vi "LogFile.vi"(7 "LogMode":T1, 8 "error in (no error)":errorcluster, 11 "LogString":string="456") -> (0 "error out":errorcluster)   [LabVIEW 2011]
uses:
  Enumerator/LogMode.ctl
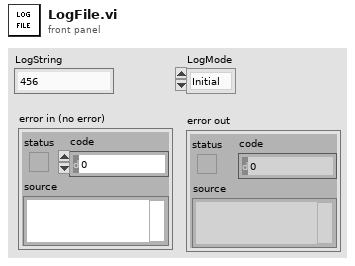
[diagram p1: front panel]
types:
  T1 = typedef "LogMode.ctl" = enum16{"Initial", "Creat", "Write", "Close"}
  T2 = enum16{"open", "replace", "create", "open or create", "replace or create", "replace or create with confirmation"}
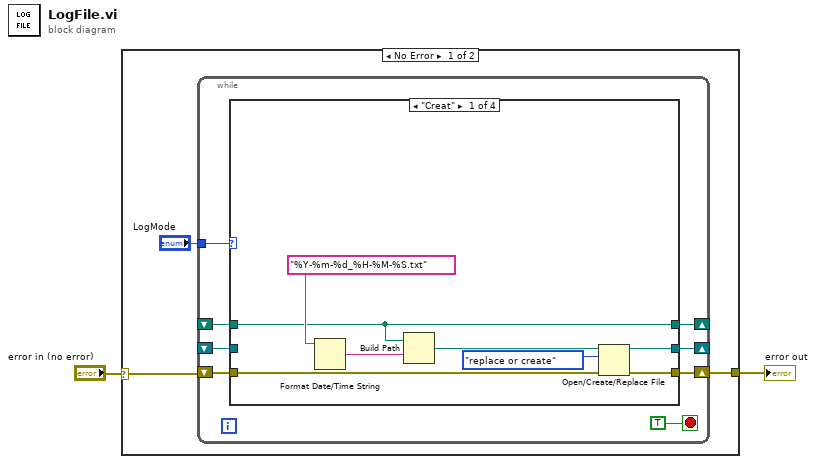
[diagram p0: block diagram]
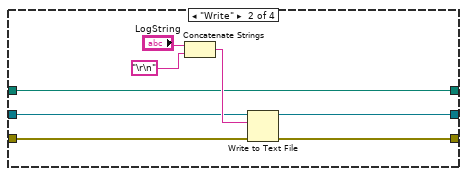
[diagram p2: hidden frame]
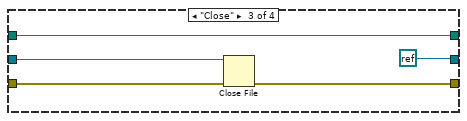
[diagram p3: hidden frame]
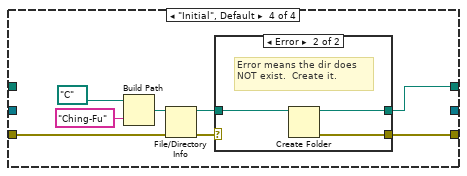
[diagram p4: hidden frame]
diagram:
  n1 = case shown="No Error" "error in (no error)" {
    selector: "error in (no error)" -> [w4 w48]
    tunnel: [w3 w48] -> w1
    frame No Error {
      n2 = while {
        shift-right: [w9] -> _
        shift-left: _ -> [w11]
        shift-right: [w10] -> _
        shift-left: _ -> [w6]
        shift-right: [w7] -> w3
        shift-left: w4 -> [w8]
        tunnel: "LogMode" -> [w13]
        stop <- TRUE stop-if-true
        n3 = case shown="\"Creat\"" w13 {
          tunnel: [w14 w22 w30 w37] -> w9
          tunnel: w11 -> [w14 w22 w30 _]
          tunnel: [w17 w23 refnum<k0> refnum _] -> w10
          tunnel: w8 -> [w16 w25 w34 w36]
          tunnel: [w15 w24 w33 w35] -> w7
          tunnel: w6 -> [_ w26 w32 _]
          frame "Creat" {
            n4 = Format Date/Time String(time format string (%c)="%Y-%m-%d_%H-%M-%S.txt") -> (date/time string=w21:string)  [unwired: 2 in]
            n5 = Build Path(base path=w14, name or relative path=w21) -> (appended path=w20:path)
            n6 = Open/Create/Replace File(file path (use dialog)=w20, error in=w16, operation (0:open)=T2."replace or create") -> (refnum out=w17:refnum<file>, error out=w15:errorcluster)  [unwired: 3 in, 1 out]
          }
          frame "Write" {
            n7 = Concatenate Strings("LogString", "\r\n") -> (w28:string)
            n8 = Write to Text File(file (use dialog)=w26, text=w28, error in=w25) -> (refnum out=w23:refnum<file>, error out=w24:errorcluster)  [unwired: 1 in, 1 out]
          }
          frame "Close" {
            n9 = Close File(refnum=w32, error in=w34) -> (error out=w33:errorcluster)  [unwired: 1 out]
          }
          frame "Initial", Default {
            n10 = Build Path(base path=path "C:/", name or relative path="Ching-Fu") -> (appended path=w39:path)
            n11 = File/Directory Info(path=w39, error in=w36) -> (path out=w41:path, error out=w40:errorcluster)  [unwired: 5 out]
            n12 = case shown="Error" w40 {
              selector: w40 -> [w43 _]
              tunnel: w41 -> [w44 w47]
              tunnel: [w44 w46] -> w37
              tunnel: [w43 w45] -> w35
              frame No Error {
                # "Directory already exists\n\nNo need to do anything"
              }
              frame Error {
                # "Error means the dir does\nNOT exist.  Create it."
                n13 = Create Folder(path (use dialog)=w47) -> (created path=w46:path, error out=w45:errorcluster)  [unwired: 2 in, 1 out]
              }
            }
          }
        }
      }
    }
    frame Error {
    }
  }
  "error out" <- w1
